vi "数字量输入.vi"(8 "CAN端口":u16, 10 "输入值":i16) -> ()   [LabVIEW 2010]
uses:
  全局量/全局_配置.vi
panel:
  out "结束？":bool
  in  "同步_2":i32
  out "数据组数":i32
  in  "同步_1":i32
  # "0或1"
  # "从1 开始"
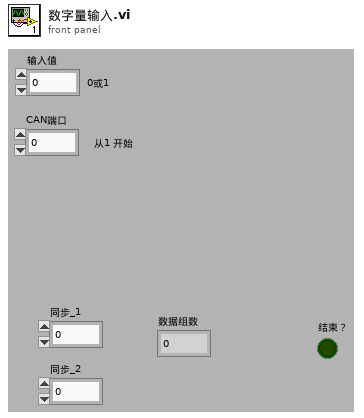
[diagram p1: front panel]
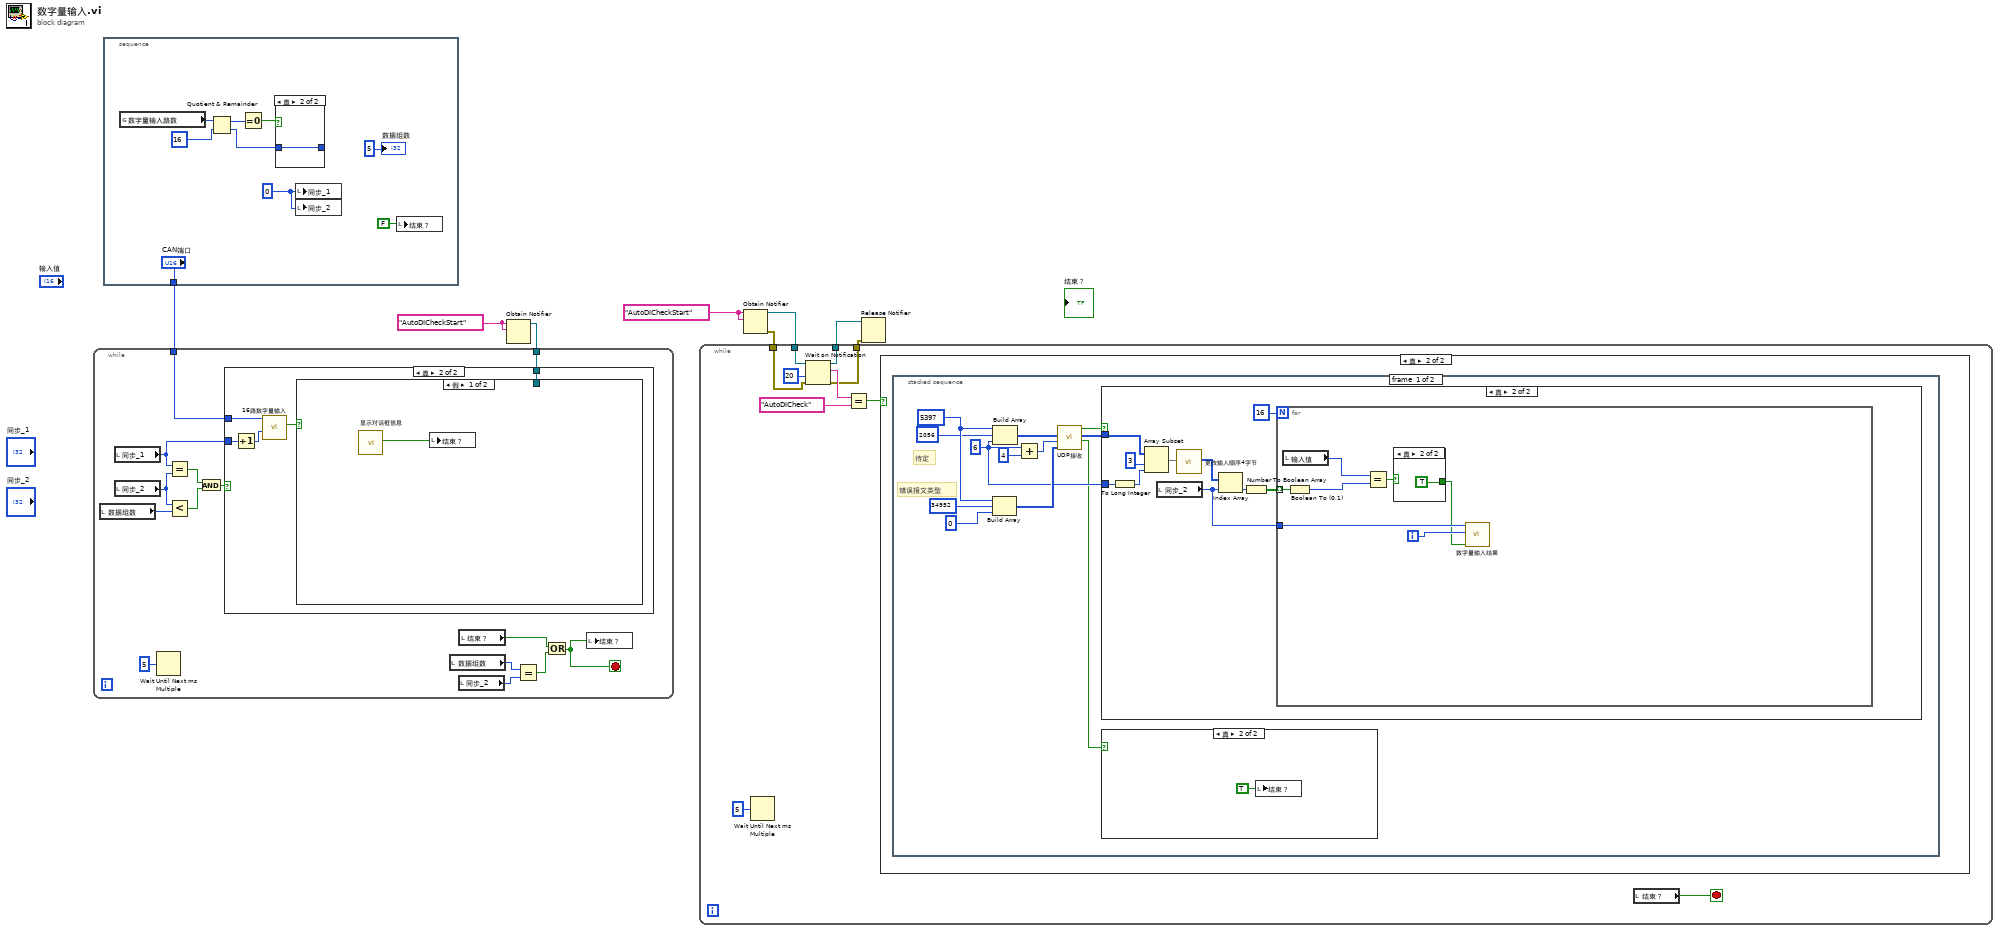
[diagram p0: block diagram]
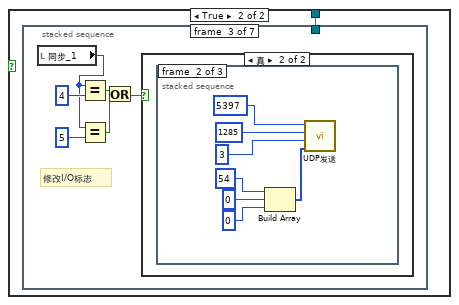
[diagram p3: hidden frame]
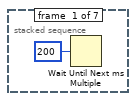
[diagram p4: hidden frame]
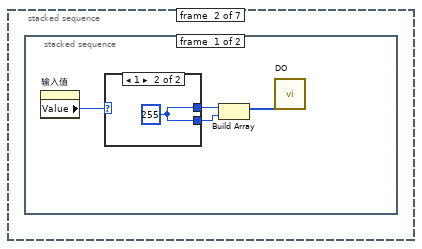
[diagram p5: hidden frame]
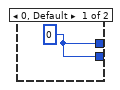
[diagram p6: hidden frame]
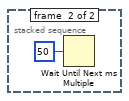
[diagram p7: hidden frame]
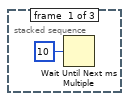
[diagram p9: hidden frame]
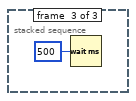
[diagram p10: hidden frame]
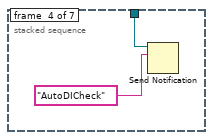
[diagram p11: hidden frame]
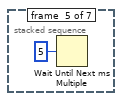
[diagram p12: hidden frame]
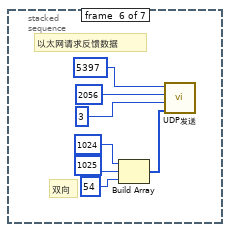
[diagram p13: hidden frame]
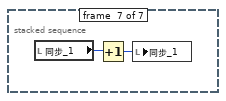
[diagram p14: hidden frame]
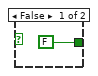
[diagram p18: hidden frame]
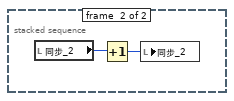
[diagram p19: hidden frame]
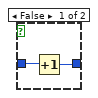
[diagram p20: hidden frame]
diagram:
  w3 = "AutoDICheckStart" ("名称（未命名）")
  w8 = "AutoDICheckStart" ("名称（未命名）")
  n1 = stacked-sequence {
    tunnel: ["CAN端口"] -> w1
    frame #0 {
      w12 = 0 ("同步_1")
      n2 = global read "全局_配置.vi" "数字量输入路数"() -> (w13:i32)
      n3 = Quotient & Remainder(x=w13, y=16) -> (x-y*floor(x/y)=w15:i32, floor(x/y)=w16:i32)
      n4 = Equal To 0?(x=w15) -> (x = 0?=w17:bool)
      n5 = case shown="真" w17 {
        tunnel: w16 -> [w19 w20]
        tunnel: [w18 w20] -> _
        frame False {
          n6 = Increment(x=w19) -> (x+1=w18:i32)
        }
        frame True {
        }
      }
      n7 = local write "同步_1"(w12) -> ()
      n8 = local write "同步_2"(w12) -> ()
      n9 = local write "结束？"(FALSE ("结束？")) -> ()
      "数据组数" <- 5 ("数据组数")
    }
  }
  n10 = Obtain Notifier(name (unnamed)=w3, notification data type=w3) -> (notifier out=w2:refnum<notifier>)  [unwired: 2 in, 2 out]
  n11 = while {
    tunnel: w2 -> [w22]
    tunnel: w1 -> [w21]
    stop <- w31 stop-if-true
    n12 = local read "数据组数"() -> (w26:i32)
    n13 = local read "同步_1"() -> (w28:i32)
    n14 = local read "同步_2"() -> (w27:i32)
    n15 = Wait Until Next ms Multiple(millisecond multiple=u32 5 ("毫秒倍数")) -> ()  [unwired: 1 out]
    n16 = Equal?(x=w28, y=w27) -> (x = y?=w24:bool)
    n17 = Less?(x=w27, y=w26) -> (x < y?=w23:bool)
    n18 = And(x=w24, y=w23) -> (x .and. y?=w25:bool)
    n19 = case shown="真" w25 {
      tunnel: w28 -> [_ w37]
      tunnel: w21 -> [_ w36]
      tunnel: w22 -> [_ w35]
      frame False {
      }
      frame True {
        n20 = Increment(x=w37) -> (x+1=w38:i32)
        n21 = call "16路数字量输入.vi"("第几组数据"=w38, "CAN端口"=w36) -> ("成功?"=w39:bool)  [unwired: 9 in]
        n22 = case shown="假" w39 {
          tunnel: w35 -> [_ w41]
          frame False {
            n23 = call "显示对话框信息"() -> ("确定"=w40:bool)  [unwired: 10 in, 1 out]
            n24 = local write "结束？"(w40) -> ()
          }
          frame True {
            n25 = stacked-sequence {
              tunnel: w41 -> [_ _ _ w65 _ _ _]
              frame #0 {
                n26 = Wait Until Next ms Multiple(millisecond multiple=u32 200 ("毫秒倍数")) -> ()  [unwired: 1 out]
              }
              frame #1 {
                n27 = stacked-sequence {
                  frame #0 {
                    n28 = property on="输入值" class="DigNum (严格)"() -> ("Value"=w43:i16)  [unwired: 2 in, 2 out]
                    n29 = case shown="1" w43 {
                      tunnel: [w47 w48] -> w45
                      tunnel: [w47 w48] -> w44
                      frame 0, Default {
                        w47 = u8 0
                      }
                      frame 1 {
                        w48 = u8 255
                      }
                    }
                    n30 = Build Array(w45, w44) -> (w46:u8[])
                    n31 = call "DO"("dataIn(U8Array)"=w46) -> ()  [unwired: 2 in, 17 out]
                  }
                  frame #1 {
                    n32 = Wait Until Next ms Multiple(millisecond multiple=u32 50 ("毫秒倍数")) -> ()  [unwired: 1 out]
                  }
                }
              }
              frame #2 {
                # "修改I/O标志"
                n33 = local read "同步_1"() -> (w51:i32)
                n34 = Equal?(x=w51, y=4) -> (x = y?=w54:bool)
                n35 = Equal?(x=w51, y=5) -> (x = y?=w55:bool)
                n36 = Or(x=w54, y=w55) -> (x .or. y?=w50:bool)
                n37 = case shown="真" w50 {
                  frame False {
                  }
                  frame True {
                    n38 = stacked-sequence {
                      frame #0 {
                        n39 = Wait Until Next ms Multiple(millisecond multiple=u32 10 ("毫秒倍数")) -> ()  [unwired: 1 out]
                      }
                      frame #1 {
                        n40 = Build Array(u16 54, u16 0, u16 0) -> (w63:u16[])
                        n41 = call "UDP发送.vi"("发送数据"=w63, "数据区字长"=u16 3, "报文类型"=u16 1285, "发送方标识"=u16 5397) -> ()  [unwired: 6 in, 1 out]
                      }
                      frame #2 {
                        n42 = Wait (ms)(milliseconds to wait=u32 500 ("毫秒倍数")) -> ()  [unwired: 1 out]
                      }
                    }
                  }
                }
              }
              frame #3 {
                n43 = Send Notification(notification="AutoDICheck" ("通知"), notifier=w65) -> ()  [unwired: 1 in, 2 out]
              }
              frame #4 {
                n44 = Wait Until Next ms Multiple(millisecond multiple=u32 5 ("等待时间（毫秒）")) -> ()  [unwired: 1 out]
              }
              frame #5 {
                # "双向"
                # "以太网请求反馈数据"
                n45 = Build Array(u16 1024, u16 1025, u16 54) -> (w69:u16[])
                n46 = call "UDP发送.vi"("发送数据"=w69, "数据区字长"=u16 3, "报文类型"=u16 2056, "发送方标识"=u16 5397) -> ()  [unwired: 6 in, 1 out]
              }
              frame #6 {
                n47 = local read "同步_1"() -> (w76:i32)
                n48 = Increment(x=w76) -> (x+1=w75:i32)
                n49 = local write "同步_1"(w75) -> ()
              }
            }
          }
        }
      }
    }
    n50 = local read "数据组数"() -> (w32:i32)
    n51 = local read "同步_2"() -> (w33:i32)
    n52 = local read "结束？"() -> (w30:bool)
    n53 = Equal?(x=w32, y=w33) -> (x = y?=w29:bool)
    n54 = Or(x=w30, y=w29) -> (x .or. y?=w31:bool)
    n55 = local write "结束？"(w31) -> ()
  }
  n56 = Obtain Notifier(name (unnamed)=w8, notification data type=w8) -> (notifier out=w7:refnum<notifier>, error out=w5:errorcluster)  [unwired: 2 in, 1 out]
  n57 = while {
    tunnel: w7 -> [w83]
    tunnel: [w82] -> w6
    tunnel: w5 -> [w81]
    tunnel: [w80] -> w4
    stop <- w78 stop-if-true
    n58 = Wait Until Next ms Multiple(millisecond multiple=u32 5 ("毫秒倍数")) -> ()  [unwired: 1 out]
    n59 = Wait on Notification(notifier=w83, timeout in ms (-1)=20 ("超时毫秒(-1)"), error in (no error)=w81) -> (notifier out=w82:refnum<notifier>, notification=w86:string, error out=w80:errorcluster)  [unwired: 1 in, 1 out]
    n60 = Equal?(x=w86, y="AutoDICheck" ("通知")) -> (x = y?=w79:bool)
    n61 = case shown="真" w79 {
      frame False {
      }
      frame True {
        n62 = stacked-sequence {
          frame #0 {
            w88 = u16 6
            w93 = u16 5397
            # "错误报文类型"
            # "待定"
            n63 = Build Array(w93, u16 34952, u16 0 ("元素")) -> (w96:u16[])
            n64 = Build Array(w93, u16 2056, w88) -> (w92:u16[])
            n65 = Add(x=w88, y=u16 4) -> (x+y=w98:u16)
            n66 = call "UDP接收.vi"("匹配帧信息_异常"=w96, "长度"=w98, "匹配帧信息_正常"=w92) -> ("接收超时?"=w87:bool, "接收的一帧数据"=w89:u16[], "正常_找到?"=w90:bool)  [unwired: 5 in, 1 out]
            n67 = case shown="真" w90 {
              tunnel: w89 -> [_ w107]
              tunnel: w88 -> [_ w106]
              frame False {
              }
              frame True {
                n68 = To Long Integer(number=w106) -> (32bit integer=w109:i32)
                n69 = Array Subset(array=w107, index=3 ("索引"), length=w109) -> (w105:u16[])
                n70 = local read "同步_2"() -> (w100:i32)
                n71 = call "更改输入顺序4字节.vi"("输入数据"=w105) -> ("更改顺序后数据"=w104:u16[])  [unwired: 10 in]
                n72 = Index Array(array=w104, index=w100) -> (element=w103:u16)
                n73 = Number To Boolean Array(number=w103) -> (Boolean array=w102:bool[])
                n74 = for {
                  N: 16 -> [_]
                  tunnel: w102 -> [w116] mode=indexing
                  tunnel: w100 -> [w112]
                  i -> [w111]
                  n75 = local read "输入值"() -> (w114:i16)
                  n76 = Boolean To (0,1)(Boolean=w116) -> (0, 1=w113:i16)
                  n77 = Equal?(x=w114, y=w113) -> (x = y?=w115:bool)
                  n78 = case shown="真" w115 {
                    tunnel: [FALSE TRUE] -> w110
                    frame False {
                    }
                    frame True {
                    }
                  }
                  n79 = call "数字量输入结果.vi"("合格?"=w110, "第几个"=w111, "第几组"=w112) -> ()  [unwired: 9 in]
                }
              }
            }
            n80 = case shown="真" w87 {
              frame False {
              }
              frame True {
                n81 = local write "结束？"(TRUE ("结束？")) -> ()
              }
            }
          }
          frame #1 {
            n82 = local read "同步_2"() -> (w120:i32)
            n83 = Increment(x=w120) -> (x+1=w119:i32)
            n84 = local write "同步_2"(w119) -> ()
          }
        }
      }
    }
    n85 = local read "结束？"() -> (w78:bool)
  }
  n86 = Release Notifier(notifier=w6, error in (no error)=w4) -> ()  [unwired: 1 in, 3 out]
